vi "Game Wizard.vi"() -> ()   [LabVIEW 2015]
uses:
  <vilib>/LAVA/UI Tools/Engine/Move Speed__lava_lib_ui_tools.ctl
  <vilib>/Utility/miscctls.llb/LVPositionTypeDef.ctl
  <vilib>/Utility/inputDevices.llb/joystickAcquire.vi
  <vilib>/Utility/inputDevices.llb/closeJoystick.vi
panel:
  in  "IP":string
  in  "Overall Help 2":bool
  out "Help 2":string
  out "Chan":i32
  out "Tab Control":T1(tab)
  in  "INIT CANCEL":bool
  in  "INIT FRONT":bool
  in  "Ch Know??":enum32{"Y", "N"}(radio)=enum."N"
  in  "CH CANCEL":bool
  in  "CH FRONT":bool
  in  "CH BK":bool
  in  "H2 CANCEL":bool
  in  "H1 FRONT":bool
  in  "H1 BK":bool
  in  "H1 CANCEL":bool
  in  "H2 FRONT":bool
  in  "H2 BK":bool
  out "Channel Being Tested":i32
  in  "H3 CANCEL":bool
  out "Final Channel":i32
  in  "H4 CANCEL":bool
  in  "H4 FRONT":bool
  in  "H4 BK":bool
  in  "H5A Skip":bool
  in  "H5A CANCEL":bool
  in  "H5A F":bool
  in  "H5A B":bool
  in  "H5B CANCEL":bool
  in  "H5B F":bool
  in  "H5B B":bool
  in  "H5C CANCEL":bool
  in  "H5C F":bool
  in  "H5C B":bool
  in  "H5D CANCEL":bool
  in  "H5D F":bool
  in  "H5D B":bool
  in  "Channel I/P":u32
  in  "TELL CANCEL":bool
  in  "TELL FRONT":bool
  in  "TELL BK":bool
  in  "Finish":bool
  # "Twin Shock Wizard"
  # "Here we will help\nyou connect to \nTwin Shock, the\ncontroller for the\nrobot"
  # "Do you know the channel??\nDo you know the channel to which\nthe Twin Shock will connect? You might\nbe knowing if you have used it earlier\nwith this very computer"
  # "Figuring out the channel: Step 1\nConnect the device to the computer via USB.\nIf this is the first time you are connecting it to\nthis PC, please let the drivers install."
  # "ILLUSTRATION ONLY"
  # "Step 2\nPlease switch the remote into Analog\nMode using the MODE button"
  # "Action Triggers"
  # "Mode\nButton"
  # "ILLUSTRATION ONLY"
  # "Please KEEP ON\n            HOLDING the \nACTION TRIGGERS till\nthe channel is identified"
  # "Please wait..\nWe are identifying the channel,\nplease give us some time"
  # "Currently testing channel"
  # "Please KEEP ON\n            HOLDING the \nACTION TRIGGERS till\nthe channel is identified"
  # "Done!!\nWe have identified the channel\nto which your remote is connected."
  # "Your remote is connected to channel no."
  # "You can now release the Action Triggers. The channel has been detected by us."
  # "Learn how to use the remote (1)\nHere we will see how to move the robot\nusing the Twin Shock game controller."
  # "ILLUSTRATION ONLY"
  # "Use these buttons or the\nDirection Pad to command\nthe robot to move"
  # "Learn how to use the remote (2)\nHere we will see how to move the meArm\nusing the Twin Shock game controller."
  # "ILLUSTRATION ONLY"
  # "The Action Triggers help jam the \narm's axis to one position:\n5  --> Base\n6  --> Shoulder\n7  --> Elbow\n8  --> Claw"
  # "Moving Joystick 1 left and\nright will control the base of\nthe arm. If you move it up\nand down, you will be moving\nthe shoulder"
  # "Moving Joystick 2 left and\nright will control the claw of\nthe arm. If you move it up\nand down, you will be moving\nthe elbow"
  # "Please be careful when using\nthe SHOULDER and the ELBOW.\nThey work together to move\nthe meArm up-down and\nfront-back"
  # "Learn how to use the remote (3)\nHere we will see how to use the special\nfunctions on the Twin Shock controller"
  # "ILLUSTRATION ONLY"
  # "These buttons have special\nfunctions in controlling\nthe robot\n1  --> Morse Out\n2  --> Camera Play\n3  --> Camera Pause\n4  --> Camera Stop"
  # "Learn how to use the remote (4)\nHere we will see how to pause the use of the\ncontroller or shut down the program altogether"
  # "ILLUSTRATION ONLY"
  # "While you are holding the\nStart Button, you cannot use\nthe controller to control the\nrobot. You can then operate\nthe buttons on the screen"
  # "Once you press the Stop\nButton on Twin Shock,\nthe program will stop runing.\nYou can use this once you are\ndone with the mission and\nwant to shut down the robot"
  # "Tell us the channel\nIn case you're aware of the channel on\nwhich this computer supports the Twin\nShock Controller, please type it here.\n\nThen plug in the controller, wait for two\nminutes, switch to Analog Mode, then\nclick NEXT"
  # "Please type in a number ONLY\neg: 0, 5, 6, 8, 3"
  # "Done!!\nYou are done with connecting Twin\nShock. Click finish to proceed on.\n\nOnce done, please double-click on\nMain myRIO (WTSS).vi. Once you\nhave the main screen, hold Ctrl and\npress R once."
  # "ILLUSTRATION ONLY"
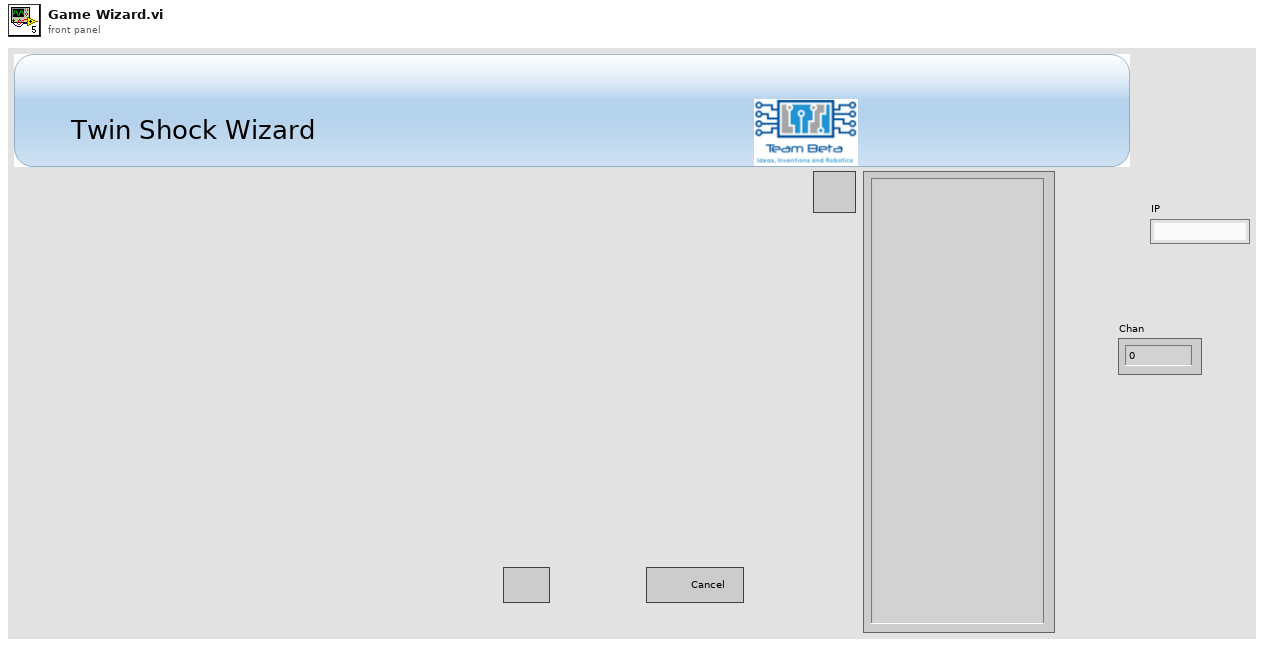
[diagram p1: front panel]
types:
  T1 = enum32{"Init", "TS Channel?", "H1", "H2", "H3", "H4", "H5A", "H5B", "H5C", "H5D", "Tell", "Done"}
  T2 = typedef "LVPositionTypeDef.ctl" = cluster{"Left":i32, "Top":i32}
  T3 = typedef "Move Speed__lava_lib_ui_tools.ctl" = enum16{"Normal", "Fast", "Slow", "Instantaneous"}
  T4 = enum32{"Invalid", "Standard", "Closed", "Hidden", "Minimized", "Maximized"}
  T5 = cluster{"button 1":bool, "button 2":bool, "button 3":bool, "button 4":bool, "button 5":bool, "button 6":bool, "button 7":bool, "button 8":bool, "button 9":bool, "button 10":bool, "button 11":bool, "button 12":bool, "button 13":bool, "button 14":bool, "button 15":bool, "button 16":bool, "button 17":bool, "button 18":bool, "button 19":bool, "button 20":bool, "button 21":bool, "button 22":bool, "button 23":bool, "button 24":bool, "button 25":bool, "button 26":bool, "button 27":bool, "button 28":bool, "button 29":bool, "button 30":bool, "button 31":bool, "button 32":bool}
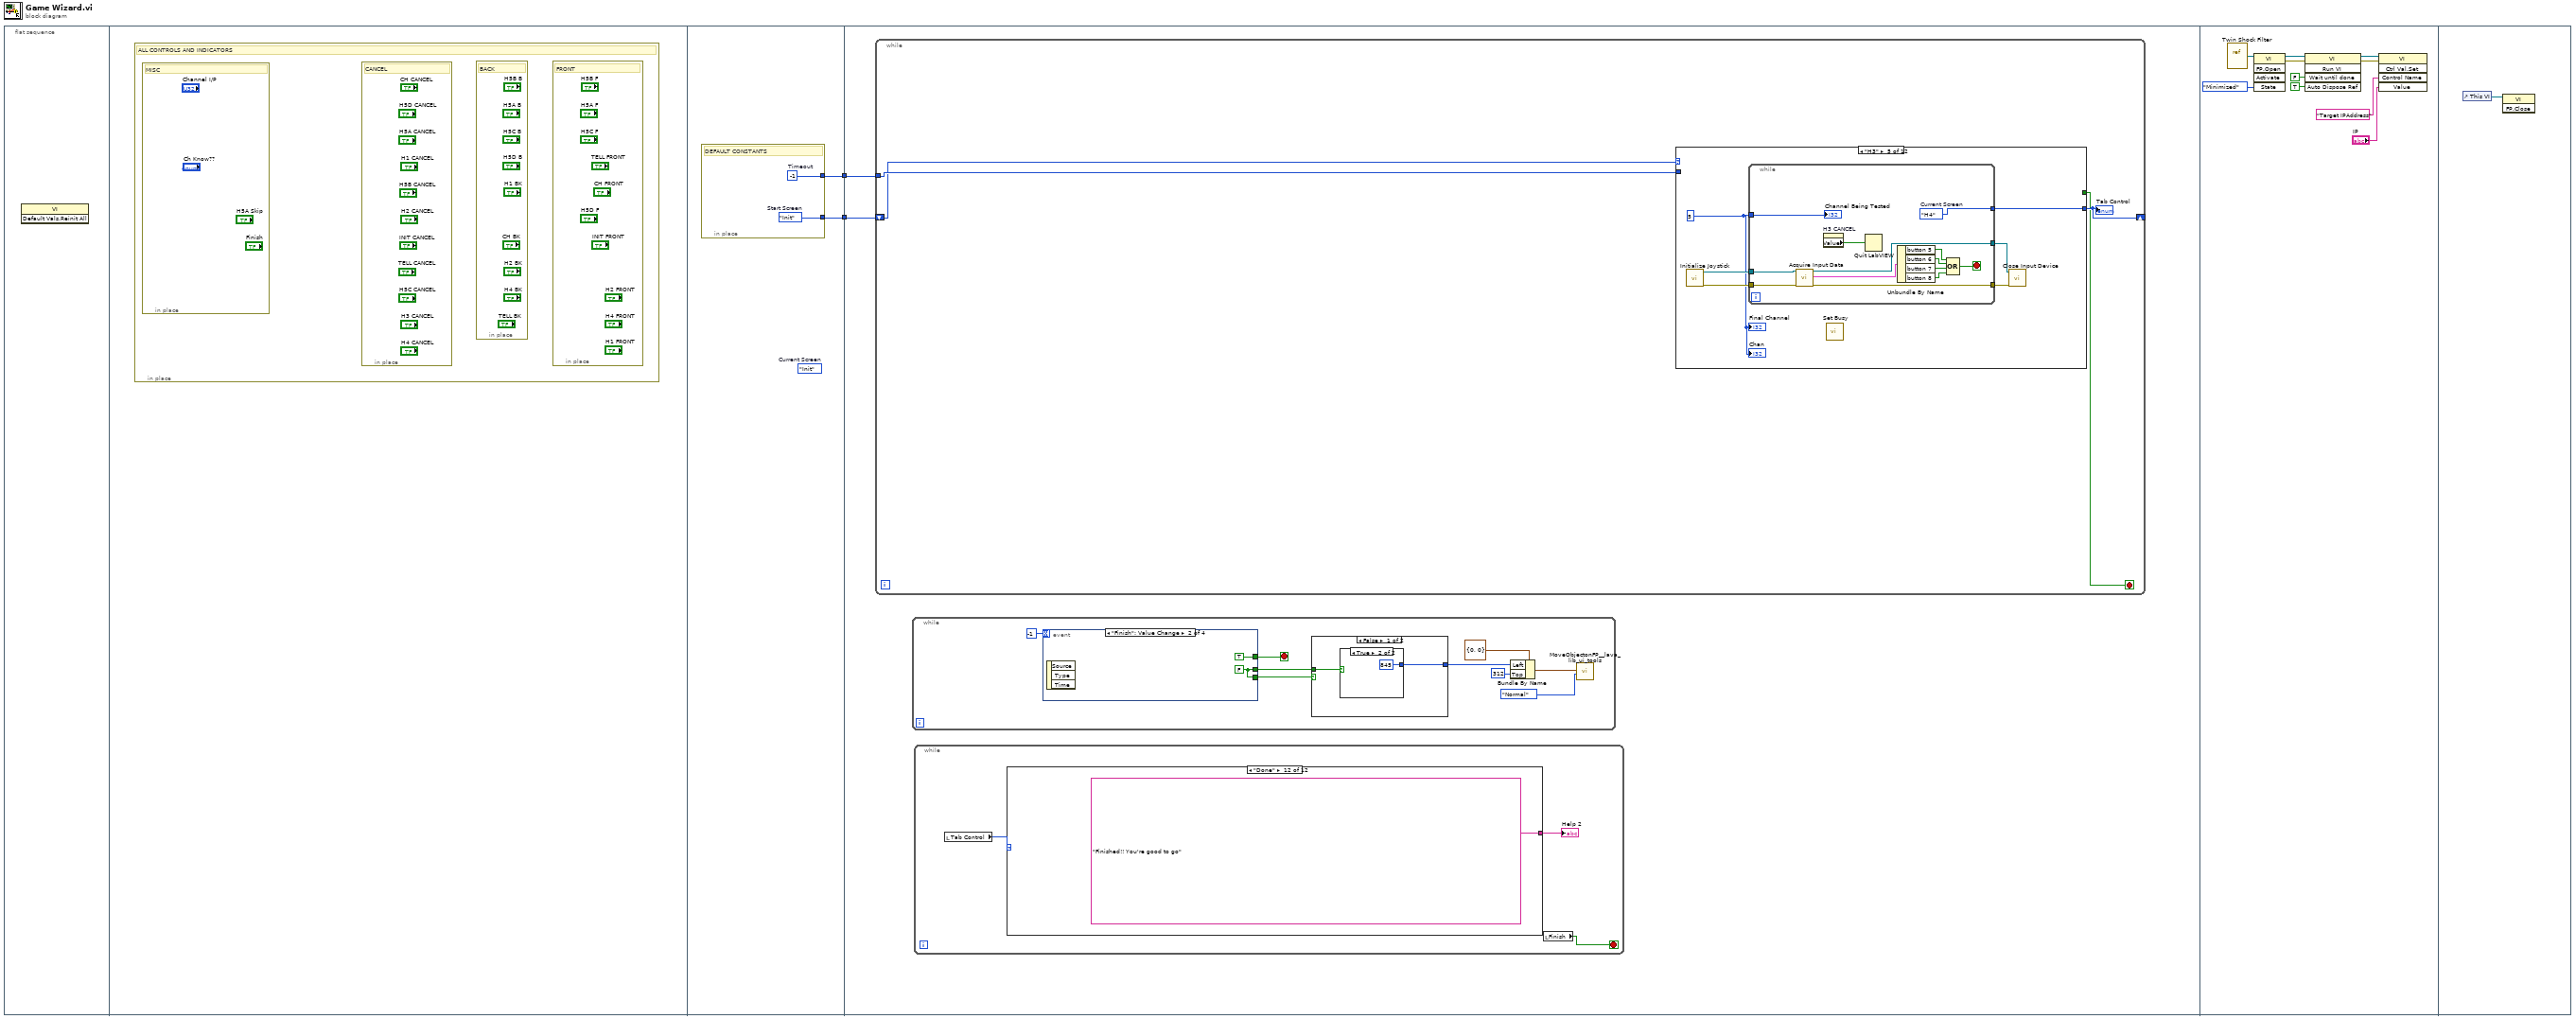
[diagram p0: block diagram]
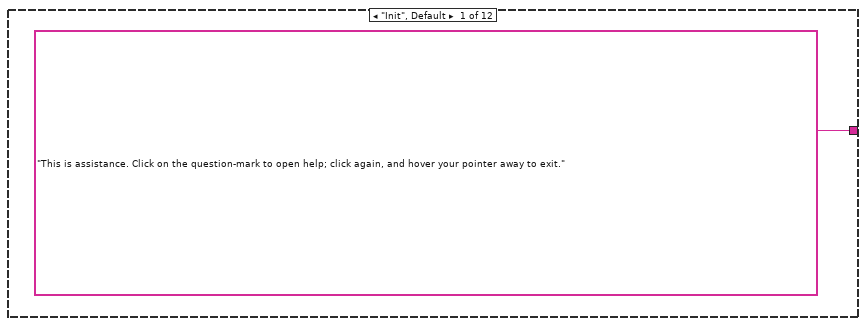
[diagram p2: hidden frame]
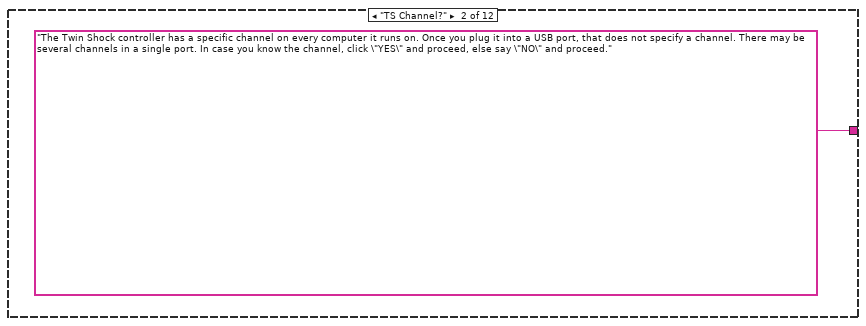
[diagram p3: hidden frame]
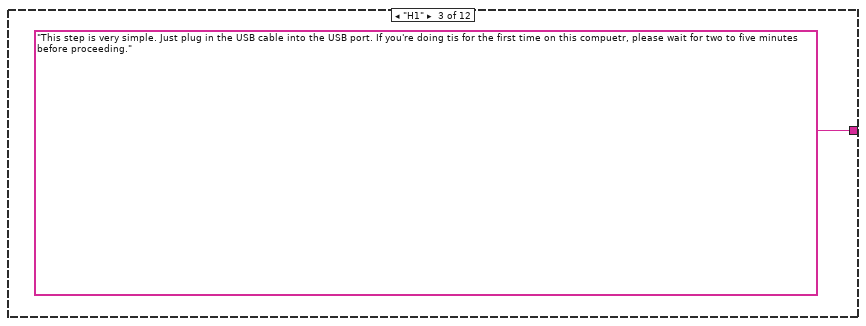
[diagram p4: hidden frame]
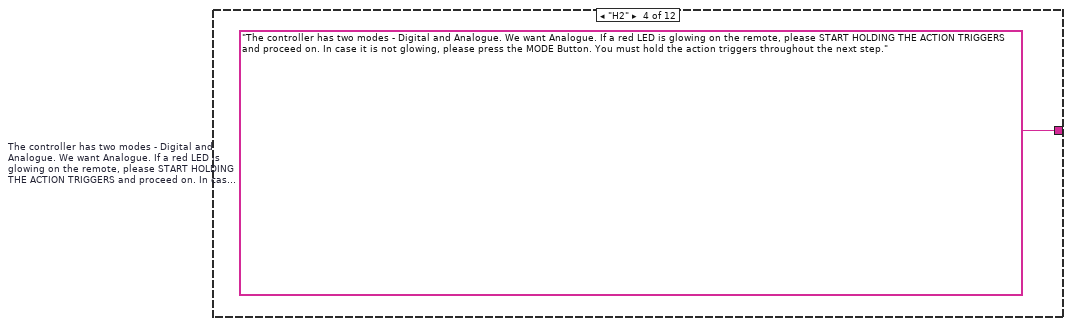
[diagram p5: hidden frame]
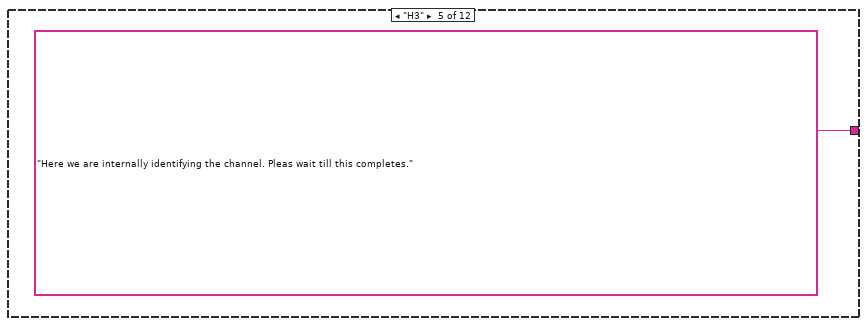
[diagram p6: hidden frame]
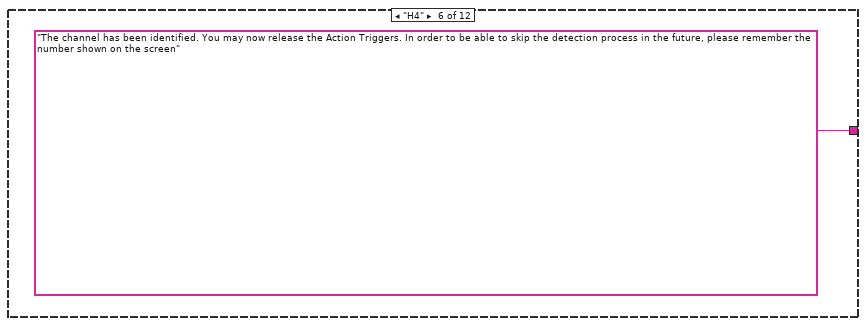
[diagram p7: hidden frame]
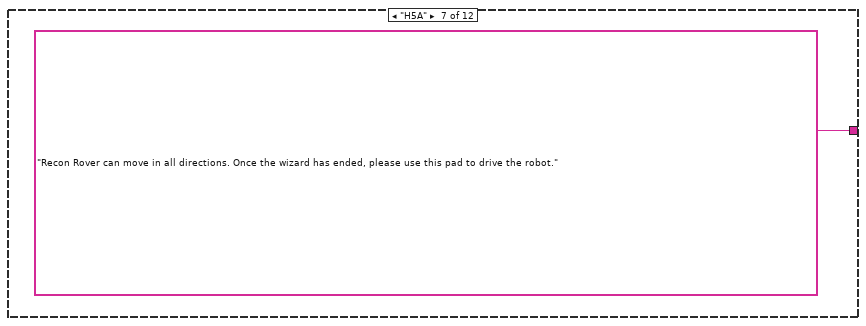
[diagram p8: hidden frame]
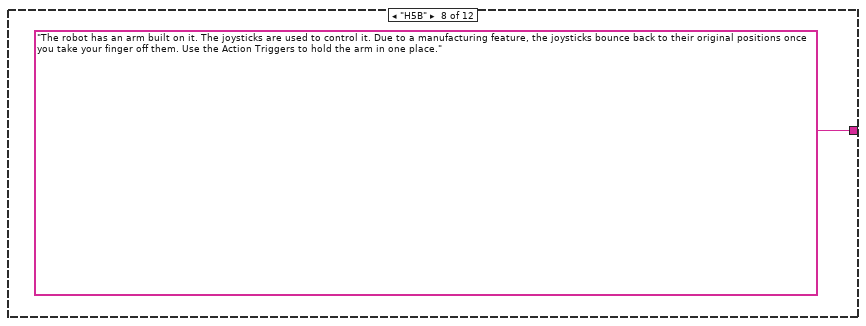
[diagram p9: hidden frame]
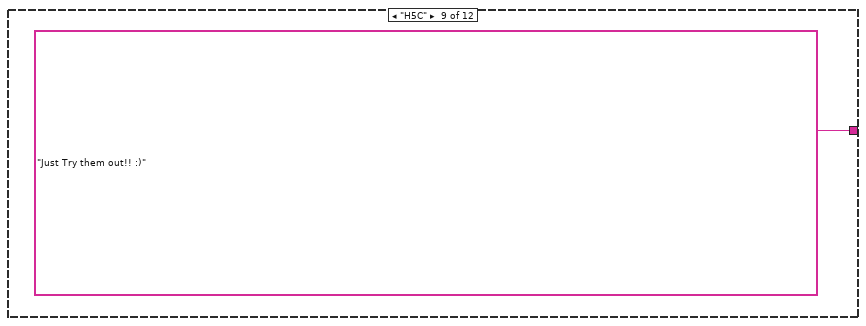
[diagram p10: hidden frame]
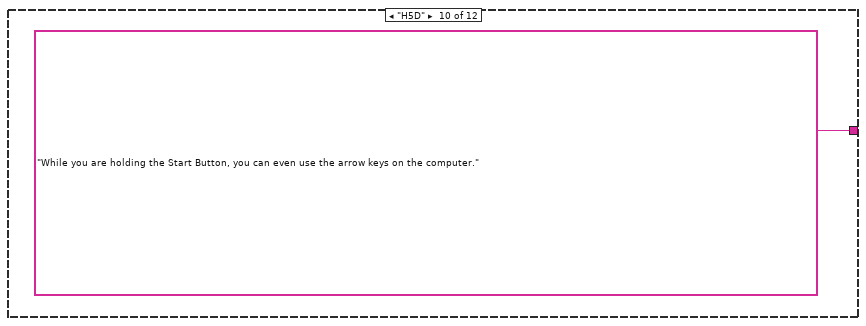
[diagram p11: hidden frame]
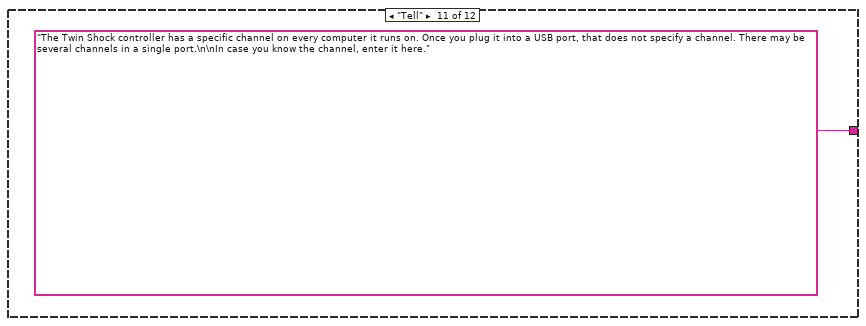
[diagram p12: hidden frame]
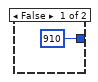
[diagram p13: hidden frame]
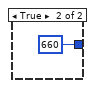
[diagram p14: hidden frame]
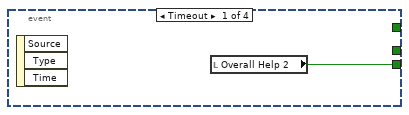
[diagram p15: hidden frame]
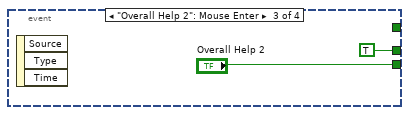
[diagram p16: hidden frame]
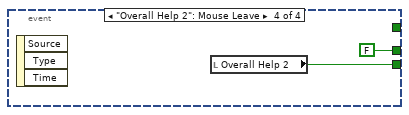
[diagram p17: hidden frame]
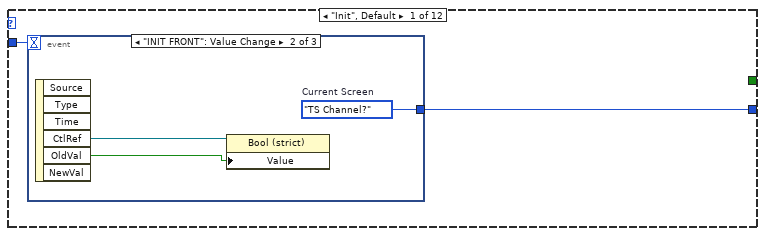
[diagram p18: hidden frame]
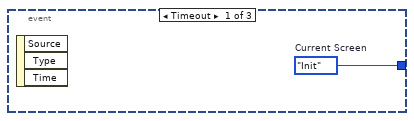
[diagram p19: hidden frame]
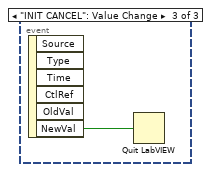
[diagram p20: hidden frame]
diagram:
  n1 = flat-sequence {
    tunnel: [w4] -> w2
    tunnel: [w3] -> w1
    tunnel: w2 -> [w8]
    tunnel: w1 -> [w7]
    frame #0 {
      n2 = invoke class="VI" method="Default Vals.Reinit All"() -> ()  [unwired: 3 in, 3 out]
    }
    frame #1 {
      n3 = in-place {
        # "ALL CONTROLS AND INDICATORS"
        n4 = in-place {
          # "MISC"
        }
        n5 = in-place {
          # "CANCEL"
        }
        n6 = in-place {
          # "BACK"
        }
        n7 = in-place {
          # "FRONT"
        }
      }
    }
    frame #2 {
      (unwired) T1."Init"  # Current Screen
      n8 = in-place {
        in-place-border: [w6] -> w4
        in-place-border: [w5] -> w3
        w5 = -1  # Timeout
        w6 = T1."Init"  # Start Screen
        # "DEFAULT CONSTANTS"
      }
    }
    frame #3 {
      n9 = while {
        shift-right: [w47] -> _
        shift-left: w8 -> [w45]
        tunnel: w7 -> [w48]
        stop <- w46 stop-if-true
        n10 = case shown="\"H3\"" w45 {
          tunnel: w48 -> [w50 w57 w70 w80 _ w109 w119 w132 w142 w152 w162 w175]
          tunnel: [w49 w56 w69 w79 w90 w108 w118 w131 w141 w151 w161 w174] -> w47
          tunnel: [_ _ _ _ _ _ _ _ _ _ _ w173] -> w46
          frame "Init", Default {
            n11 = event shown="[1] \"INIT FRONT\": Value Change" {
              selector: _ -> [_ _ _]
              dyn-events: _ -> [_ _ _]
              timeout: w50 -> [_ _ _]
              tunnel: [w51 w54 _] -> w49
              event Timeout {
                w51 = T1."Init"  # Current Screen
                n12 = event-data() -> ()  [unwired: 1 in, 3 out]
              }
              event "INIT FRONT": Value Change {
                w54 = T1."TS Channel?"  # Current Screen
                n13 = event-data() -> ("CtlRef"=w53:refnum<vi>, "OldVal"=w52:bool)  [unwired: 1 in, 4 out]
                n14 = property class="Bool (strict)"(reference=w53, "Value"=w52) -> ()  [unwired: 1 in, 2 out]
              }
              event "INIT CANCEL": Value Change {
                n15 = event-data() -> ("NewVal"=w55:bool)  [unwired: 1 in, 5 out]
                n16 = Quit LabVIEW(quit? (T)=w55) -> ()
              }
            }
          }
          frame "TS Channel?" {
            n17 = event shown="[0] Timeout" {
              selector: _ -> [_ _ _ _]
              dyn-events: _ -> [_ _ _ _]
              timeout: w57 -> [_ _ _ _]
              tunnel: [w58 w59 w67 _] -> w56
              event Timeout {
                w58 = T1."TS Channel?"  # Current Screen
                n18 = event-data() -> ()  [unwired: 1 in, 3 out]
              }
              event "CH FRONT": Value Change {
                n19 = event-data() -> ("CtlRef"=w62:refnum<vi>, "OldVal"=w61:bool)  [unwired: 1 in, 4 out]
                n20 = local read "Ch Know??"() -> (w60:enum32{"Y", "N"})
                n21 = property class="Bool (strict)"(reference=w62, "Value"=w61) -> ()  [unwired: 1 in, 2 out]
                n22 = case shown="\"Y\", Default" w60 {
                  tunnel: [w63 w64] -> w59
                  frame "Y", Default {
                    w63 = T1."Tell"  # Current Screen
                  }
                  frame "N" {
                    w64 = T1."H1"  # Current Screen
                  }
                }
              }
              event "CH BK": Value Change {
                w67 = T1."Init"  # Current Screen
                n23 = event-data() -> ("CtlRef"=w66:refnum<vi>, "OldVal"=w65:bool)  [unwired: 1 in, 4 out]
                n24 = property class="Bool (strict)"(reference=w66, "Value"=w65) -> ()  [unwired: 1 in, 2 out]
              }
              event "CH CANCEL": Value Change {
                n25 = event-data() -> ("NewVal"=w68:bool)  [unwired: 1 in, 5 out]
                n26 = Quit LabVIEW(quit? (T)=w68) -> ()
              }
            }
          }
          frame "H1" {
            n27 = event shown="[2] \"H1 BK\": Value Change" {
              selector: _ -> [_ _ _ _]
              dyn-events: _ -> [_ _ _ _]
              timeout: w70 -> [_ _ _ _]
              tunnel: [w71 w72 w77 _] -> w69
              event Timeout {
                w71 = T1."H1"  # Current Screen
                n28 = event-data() -> ()  [unwired: 1 in, 3 out]
              }
              event "H1 FRONT": Value Change {
                w72 = T1."H2"  # Current Screen
                n29 = event-data() -> ("CtlRef"=w74:refnum<vi>, "OldVal"=w73:bool)  [unwired: 1 in, 4 out]
                n30 = property class="Bool (strict)"(reference=w74, "Value"=w73) -> ()  [unwired: 1 in, 2 out]
              }
              event "H1 BK": Value Change {
                w77 = T1."TS Channel?"  # Current Screen
                n31 = event-data() -> ("CtlRef"=w76:refnum<vi>, "OldVal"=w75:bool)  [unwired: 1 in, 4 out]
                n32 = property class="Bool (strict)"(reference=w76, "Value"=w75) -> ()  [unwired: 1 in, 2 out]
              }
              event "H1 CANCEL": Value Change {
                n33 = event-data() -> ("NewVal"=w78:bool)  [unwired: 1 in, 5 out]
                n34 = Quit LabVIEW(quit? (T)=w78) -> ()
              }
            }
          }
          frame "H2" {
            n35 = event shown="[1] \"H2 FRONT\": Value Change" {
              selector: _ -> [_ _ _ _]
              dyn-events: _ -> [_ _ _ _]
              timeout: w80 -> [_ _ _ _]
              tunnel: [w81 w82 w87 _] -> w79
              event Timeout {
                w81 = T1."H2"  # Current Screen
                n36 = event-data() -> ()  [unwired: 1 in, 3 out]
              }
              event "H2 FRONT": Value Change {
                w82 = T1."H3"  # Current Screen
                n37 = event-data() -> ("CtlRef"=w84:refnum<vi>, "OldVal"=w83:bool)  [unwired: 1 in, 4 out]
                n38 = property class="Bool (strict)"(reference=w84, "Value"=w83) -> ()  [unwired: 1 in, 2 out]
              }
              event "H2 BK": Value Change {
                w87 = T1."H1"  # Current Screen
                n39 = event-data() -> ("CtlRef"=w86:refnum<vi>, "OldVal"=w85:bool)  [unwired: 1 in, 4 out]
                n40 = property class="Bool (strict)"(reference=w86, "Value"=w85) -> ()  [unwired: 1 in, 2 out]
              }
              event "H2 CANCEL": Value Change {
                n41 = event-data() -> ("NewVal"=w88:bool)  [unwired: 1 in, 5 out]
                n42 = Quit LabVIEW(quit? (T)=w88) -> ()
              }
            }
          }
          frame "H3" {
            w89 = 5 ("Channel Being Tested")
            n43 = call <vilib>:"Initialize Joystick.vi"() -> ("error out"=w93:errorcluster, "device ID"=w94:refnum<k1>)  [unwired: 10 in]
            n44 = while {
              tunnel: w94 -> [w106]
              tunnel: w93 -> [w105]
              tunnel: [w104] -> w92
              tunnel: [w103] -> w91
              tunnel: [w96] -> w90
              tunnel: w89 -> [w95]
              stop <- w97 stop-if-true
              w96 = T1."H4"  # Current Screen
              n45 = call-poly <vilib>:"Acquire Input Data.vi"("device ID"=w106, "error in (no error)"=w105) -> ("device ID"=w104:refnum<k1>, "button info"=w102:T5, "error out"=w103:errorcluster)  [unwired: 13 in, 2 out]
              n46 = property on="H3 CANCEL" class="Bool (strict)"() -> ("Value"=w107:bool)  [unwired: 2 in, 2 out]
              n47 = Quit LabVIEW(quit? (T)=w107) -> ()
              n48 = Unbundle By Name(w102) -> ("button 5"=w101:bool, "button 6"=w100:bool, "button 7"=w99:bool, "button 8"=w98:bool)
              n49 = Compound Arithmetic op=OR(w101, w100, w99, w98) -> (w97:bool)
              "Channel Being Tested" <- w95
            }
            n50 = call <vilib>:"Set Busy.vi"() -> ()  [unwired: 10 in, 2 out]
            n51 = call-poly <vilib>:"Close Input Device.vi"("error in (no error)"=w91, "device ID"=w92) -> ()  [unwired: 8 in, 1 out]
            "Chan" <- w89
            "Final Channel" <- w89
          }
          frame "H4" {
            n52 = event shown="[1] \"H4 FRONT\": Value Change" {
              selector: _ -> [_ _ _ _]
              dyn-events: _ -> [_ _ _ _]
              timeout: w109 -> [_ _ _ _]
              tunnel: [w110 w111 w116 _] -> w108
              event Timeout {
                w110 = T1."H4"  # Current Screen
                n53 = event-data() -> ()  [unwired: 1 in, 3 out]
              }
              event "H4 FRONT": Value Change {
                w111 = T1."H5A"  # Current Screen
                n54 = event-data() -> ("CtlRef"=w113:refnum<vi>, "OldVal"=w112:bool)  [unwired: 1 in, 4 out]
                n55 = property class="Bool (strict)"(reference=w113, "Value"=w112) -> ()  [unwired: 1 in, 2 out]
              }
              event "H4 BK": Value Change {
                w116 = T1."H3"  # Current Screen
                n56 = event-data() -> ("CtlRef"=w115:refnum<vi>, "OldVal"=w114:bool)  [unwired: 1 in, 4 out]
                n57 = property class="Bool (strict)"(reference=w115, "Value"=w114) -> ()  [unwired: 1 in, 2 out]
              }
              event "H4 CANCEL": Value Change {
                n58 = event-data() -> ("NewVal"=w117:bool)  [unwired: 1 in, 5 out]
                n59 = Quit LabVIEW(quit? (T)=w117) -> ()
              }
            }
            n60 = call <vilib>:"Unset Busy.vi"() -> ()  [unwired: 11 in, 1 out]
          }
          frame "H5A" {
            n61 = event shown="[1] \"H5A F\": Value Change" {
              selector: _ -> [_ _ _ _ _]
              dyn-events: _ -> [_ _ _ _ _]
              timeout: w119 -> [_ _ _ _ _]
              tunnel: [w120 w121 w124 w129 _] -> w118
              event Timeout {
                w120 = T1."H5A"  # Current Screen
                n62 = event-data() -> ()  [unwired: 1 in, 3 out]
              }
              event "H5A F": Value Change {
                w121 = T1."H5B"  # Current Screen
                n63 = event-data() -> ("CtlRef"=w123:refnum<vi>, "OldVal"=w122:bool)  [unwired: 1 in, 4 out]
                n64 = property class="Bool (strict)"(reference=w123, "Value"=w122) -> ()  [unwired: 1 in, 2 out]
              }
              event "H5A Skip": Value Change {
                w124 = T1."Done"  # Current Screen
                n65 = event-data() -> ("CtlRef"=w126:refnum<vi>, "OldVal"=w125:bool)  [unwired: 1 in, 4 out]
                n66 = property class="Bool (strict)"(reference=w126, "Value"=w125) -> ()  [unwired: 1 in, 2 out]
              }
              event "H5A B": Value Change {
                w129 = T1."H4"  # Current Screen
                n67 = event-data() -> ("CtlRef"=w128:refnum<vi>, "OldVal"=w127:bool)  [unwired: 1 in, 4 out]
                n68 = property class="Bool (strict)"(reference=w128, "Value"=w127) -> ()  [unwired: 1 in, 2 out]
              }
              event "H5A CANCEL": Value Change {
                n69 = event-data() -> ("NewVal"=w130:bool)  [unwired: 1 in, 5 out]
                n70 = Quit LabVIEW(quit? (T)=w130) -> ()
              }
            }
          }
          frame "H5B" {
            n71 = event shown="[1] \"H5B F\": Value Change" {
              selector: _ -> [_ _ _ _]
              dyn-events: _ -> [_ _ _ _]
              timeout: w132 -> [_ _ _ _]
              tunnel: [w133 w134 w139 _] -> w131
              event Timeout {
                w133 = T1."H5B"  # Current Screen
                n72 = event-data() -> ()  [unwired: 1 in, 3 out]
              }
              event "H5B F": Value Change {
                w134 = T1."H5C"  # Current Screen
                n73 = event-data() -> ("CtlRef"=w136:refnum<vi>, "OldVal"=w135:bool)  [unwired: 1 in, 4 out]
                n74 = property class="Bool (strict)"(reference=w136, "Value"=w135) -> ()  [unwired: 1 in, 2 out]
              }
              event "H5B B": Value Change {
                w139 = T1."H5A"  # Current Screen
                n75 = event-data() -> ("CtlRef"=w138:refnum<vi>, "OldVal"=w137:bool)  [unwired: 1 in, 4 out]
                n76 = property class="Bool (strict)"(reference=w138, "Value"=w137) -> ()  [unwired: 1 in, 2 out]
              }
              event "H5B CANCEL": Value Change {
                n77 = event-data() -> ("NewVal"=w140:bool)  [unwired: 1 in, 5 out]
                n78 = Quit LabVIEW(quit? (T)=w140) -> ()
              }
            }
          }
          frame "H5C" {
            n79 = event shown="[1] \"H5C F\": Value Change" {
              selector: _ -> [_ _ _ _]
              dyn-events: _ -> [_ _ _ _]
              timeout: w142 -> [_ _ _ _]
              tunnel: [w143 w144 w149 _] -> w141
              event Timeout {
                w143 = T1."H5C"  # Current Screen
                n80 = event-data() -> ()  [unwired: 1 in, 3 out]
              }
              event "H5C F": Value Change {
                w144 = T1."H5D"  # Current Screen
                n81 = event-data() -> ("CtlRef"=w146:refnum<vi>, "OldVal"=w145:bool)  [unwired: 1 in, 4 out]
                n82 = property class="Bool (strict)"(reference=w146, "Value"=w145) -> ()  [unwired: 1 in, 2 out]
              }
              event "H5C B": Value Change {
                w149 = T1."H5B"  # Current Screen
                n83 = event-data() -> ("CtlRef"=w148:refnum<vi>, "OldVal"=w147:bool)  [unwired: 1 in, 4 out]
                n84 = property class="Bool (strict)"(reference=w148, "Value"=w147) -> ()  [unwired: 1 in, 2 out]
              }
              event "H5C CANCEL": Value Change {
                n85 = event-data() -> ("NewVal"=w150:bool)  [unwired: 1 in, 5 out]
                n86 = Quit LabVIEW(quit? (T)=w150) -> ()
              }
            }
          }
          frame "H5D" {
            n87 = event shown="[1] \"H5D F\": Value Change" {
              selector: _ -> [_ _ _ _]
              dyn-events: _ -> [_ _ _ _]
              timeout: w152 -> [_ _ _ _]
              tunnel: [w153 w154 w159 _] -> w151
              event Timeout {
                w153 = T1."H5D"  # Current Screen
                n88 = event-data() -> ()  [unwired: 1 in, 3 out]
              }
              event "H5D F": Value Change {
                w154 = T1."Done"  # Current Screen
                n89 = event-data() -> ("CtlRef"=w156:refnum<vi>, "OldVal"=w155:bool)  [unwired: 1 in, 4 out]
                n90 = property class="Bool (strict)"(reference=w156, "Value"=w155) -> ()  [unwired: 1 in, 2 out]
              }
              event "H5D B": Value Change {
                w159 = T1."H5C"  # Current Screen
                n91 = event-data() -> ("CtlRef"=w158:refnum<vi>, "OldVal"=w157:bool)  [unwired: 1 in, 4 out]
                n92 = property class="Bool (strict)"(reference=w158, "Value"=w157) -> ()  [unwired: 1 in, 2 out]
              }
              event "H5D CANCEL": Value Change {
                n93 = event-data() -> ("NewVal"=w160:bool)  [unwired: 1 in, 5 out]
                n94 = Quit LabVIEW(quit? (T)=w160) -> ()
              }
            }
          }
          frame "Tell" {
            n95 = event shown="[3] \"TELL CANCEL\": Value Change" {
              selector: _ -> [_ _ _ _]
              dyn-events: _ -> [_ _ _ _]
              timeout: w162 -> [_ _ _ _]
              tunnel: [w163 w166 w169 _] -> w161
              event Timeout {
                w163 = T1."Tell"  # Current Screen
                n96 = event-data() -> ()  [unwired: 1 in, 3 out]
              }
              event "TELL FRONT": Value Change {
                w166 = T1."Done"  # Current Screen
                n97 = event-data() -> ("CtlRef"=w168:refnum<vi>, "OldVal"=w167:bool)  [unwired: 1 in, 4 out]
                n98 = property on="Channel I/P" class="DigNum (strict)"() -> (error out=w165:errorcluster, "Value"=w164:u32)  [unwired: 2 in, 1 out]
                n99 = property class="Bool (strict)"(reference=w168, "Value"=w167) -> ()  [unwired: 1 in, 2 out]
                n100 = property on="Chan" class="DigNum (strict)"(error in=w165, "Value"=w164) -> ()  [unwired: 1 in, 2 out]
              }
              event "TELL BK": Value Change {
                w169 = T1."TS Channel?"  # Current Screen
                n101 = event-data() -> ("CtlRef"=w171:refnum<vi>, "OldVal"=w170:bool)  [unwired: 1 in, 4 out]
                n102 = property class="Bool (strict)"(reference=w171, "Value"=w170) -> ()  [unwired: 1 in, 2 out]
              }
              event "TELL CANCEL": Value Change {
                n103 = event-data() -> ("NewVal"=w172:bool)  [unwired: 1 in, 5 out]
                n104 = Quit LabVIEW(quit? (T)=w172) -> ()
              }
            }
          }
          frame "Done" {
            n105 = event shown="[0] Timeout" {
              selector: _ -> [_ _]
              dyn-events: _ -> [_ _]
              timeout: w175 -> [_ _]
              tunnel: [w177 w179] -> w174
              tunnel: [FALSE TRUE] -> w173
              event Timeout {
                w177 = T1."Tell"  # Current Screen
                n106 = event-data() -> ()  [unwired: 1 in, 3 out]
              }
              event "Finish": Value Change {
                w179 = T1."Done"  # Current Screen
                n107 = event-data() -> ("CtlRef"=w181:refnum<vi>, "OldVal"=w180:bool)  [unwired: 1 in, 4 out]
                n108 = property class="Bool (strict)"(reference=w181, "Value"=w180) -> ()  [unwired: 1 in, 2 out]
              }
            }
          }
        }
        "Tab Control" <- w47
      }
      n109 = while {
        stop <- w31 stop-if-true
        n110 = event shown="[1] \"Finish\": Value Change" {
          selector: _ -> [_ _ _ _]
          dyn-events: _ -> [_ _ _ _]
          timeout: -1 -> [_ _ _ _]
          tunnel: [_ w39 TRUE FALSE] -> w29
          tunnel: [w38 w39 "Overall Help 2" w43] -> w28
          tunnel: [_ TRUE ("Stop Button") _ _] -> w31
          event Timeout {
            n111 = event-data() -> ()  [unwired: 1 in, 3 out]
            n112 = local read "Overall Help 2"() -> (w38:bool)
          }
          event "Finish": Value Change {
            w39 = FALSE
            n113 = event-data() -> ()  [unwired: 1 in, 3 out]
          }
          event "Overall Help 2": Mouse Enter {
            n114 = event-data() -> ()  [unwired: 1 in, 3 out]
          }
          event "Overall Help 2": Mouse Leave {
            n115 = event-data() -> ()  [unwired: 1 in, 3 out]
            n116 = local read "Overall Help 2"() -> (w43:bool)
          }
        }
        n117 = case shown="False" w28 {
          tunnel: w29 -> [w34 _]
          tunnel: [w33 660] -> w24
          frame False {
            n118 = case shown="True" w34 {
              tunnel: [910 845] -> w33
              frame False {
              }
              frame True {
              }
            }
          }
          frame True {
          }
        }
        n119 = Bundle By Name(cluster=T2 {"Left"=0, "Top"=0} ("Center Position for Object"), "Left"=w24, "Top"=312) -> (w25:T2)
        n120 = call <vilib>:"MoveObjectonFP__lava_lib_ui_tools.vi"("Move Speed (Instantaneous)"=Move_Speed__lava_lib_ui_tools."Normal", "Center Position for Object"=w25) -> ()  [unwired: 8 in, 2 out]
      }
      n121 = while {
        stop <- w11 stop-if-true
        n122 = local read "Tab Control"() -> (w10:T1)
        n123 = case shown="\"Done\"" w10 {
          tunnel: ["This is assistance. Click on the question-mark to open help; click again, and hover your pointer away to exit." "The Twin Shock controller has a specific channel on every computer it runs on. Once you plug it into a USB port, that does not specify a channel. There may be several channels in a single port. In case you know the channel, click \"YES\" and proceed, else say \"NO\" and proceed." "This step is very simple. Just plug in the USB cable into the USB port. If you're doing tis for the first time on this compuetr, please wait for two to five minutes before proceeding." w15 "Here we are internally identifying the channel. Pleas wait till this completes." "The channel has been identified. You may now release the Action Triggers. In order to be able to skip the detection process in the future, please remember the number shown on the screen" "Recon Rover can move in all directions. Once the wizard has ended, please use this pad to drive the robot." "The robot has an arm built on it. The joysticks are used to control it. Due to a manufacturing feature, the joysticks bounce back to their original positions once you take your finger off them. Use the Action Triggers to hold the arm in one place." "Just Try them out!! :)" "While you are holding the Start Button, you can even use the arrow keys on the computer." "The Twin Shock controller has a specific channel on every computer it runs on. Once you plug it into a USB port, that does not specify a channel. There may be several channels in a single port.\n\nIn case you know the channel, enter it here." "Finished!! You're good to go"] -> w9
          frame "Init", Default {
          }
          frame "TS Channel?" {
          }
          frame "H1" {
          }
          frame "H2" {
            w15 = "The controller has two modes - Digital and Analogue. We want Analogue. If a red LED is glowing on the remote, please START HOLDING THE ACTION TRIGGERS and proceed on. In case it is not glowing, please press the MODE Button. You must hold the action triggers throughout the next step."  # The controller has two modes - Digital and Analogue. We want Analogue. If a red LED is glowing on the remote, please START HOLDING THE ACTION TRIGGERS and proceed on. In case it is not glowing, please press the MODE Button. You must hold the action triggers throughout the next step.
          }
          frame "H3" {
          }
          frame "H4" {
          }
          frame "H5A" {
          }
          frame "H5B" {
          }
          frame "H5C" {
          }
          frame "H5D" {
          }
          frame "Tell" {
          }
          frame "Done" {
          }
        }
        "Help 2" <- w9
        n124 = local read "Finish"() -> (w11:bool)
      }
    }
    frame #4 {
      n125 = vi-ref "Twin Shock Filter.vi"() -> (w191:refnum<vi>)
      n126 = invoke class="VI" method="FP.Open"(reference=w191, "State"=T4."Minimized") -> (reference out=w185:refnum<vi>, error out=w184:errorcluster)  [unwired: 3 in, 3 out]
      n127 = invoke class="VI" method="Run VI"(reference=w185, error in=w184, "Wait until done"=FALSE ("Wait Until Done"), "Auto Dispose Ref"=TRUE ("Auto Dispose Reference")) -> (reference out=w183:refnum<vi>, error out=w182:errorcluster)  [unwired: 1 in, 3 out]
      n128 = invoke class="VI" method="Ctrl Val.Set"(reference=w183, error in=w182, "Control Name"="Target IPAddress", "Value"="IP") -> ()  [unwired: 1 in, 5 out]
    }
    frame #5 {
      n129 = control-ref of="This VI"() -> (w192:refnum<vi>)
      n130 = invoke class="VI" method="FP.Close"(reference=w192) -> ()  [unwired: 2 in, 3 out]
    }
  }
